vi "Configure.vi"(8 "error in":errorcluster, 10 "name":string="cCRDS", 11 "cCRDS in":refnum<class "cCRDS.lvclass">=refnum) -> (0 "error out":errorcluster, 3 "cCRDS out":refnum<class "cCRDS.lvclass">)   [LabVIEW 2015, in "cCRDS.lvclass"]
doc: "By far, the most complex of cCRDS VIs. This override of the Instrument Configure VI configures all signal input and output. The configuration is kicked off by calling the parent which sets up queues and names gives the class a unique name. Each CRDS class contains a CRDS Cell class which will encapsulate all of the defining characteristics of the discrete cell including how calculations are performed and the r factor (Optical Time Constant). In this case, each CRDS cell shares the same attributes aside from the wavelength of light used by the cavity.\n\nAfter the properties of the class are defined, the DAQmx tasks are configured. In this implementation, the CRDS utilizes two different laser types for light sources in the cavities: a dioed which requires a ring up time and a YAG which introduces light in pulses. Both laser sources (there are actually two diodes, red and blue, and one YAG, green) are fired using counter outputs. The YAG is synced with the diode counter by triggering the start of generation on the falling edge of the diode signal. On the laser acquisition side, the signal from the photodiodes is collected at a rate of 2.5 MS/s/ch using an S-series card. The acquisition signal is gated using the YAG counter signal which is tied to a counter on the S-series card across the PXI backplane using PXI_Trig0. The AI is acquired continuously clocking off of the other counter on the S-series card which is gated by the first counter.\n\nIn addition, the lasers and humidifier TECs are enabled and the humidifiers are set to their coldest temperature (corresponding to 5 V). All tasks are aggregated into a single array and started. If an error is thrown at config time, then the system will be shutdown."
uses:
  cCRDS.lvclass
  Data/cCRDS Data.lvclass
  Reusable/CRDS/Data/Cell/CRDS Cell Data.lvclass
  Reusable/CRDS/Main/CRDS.lvclass/CRDS.ctl
  Reusable/Instrument/Instrument.lvclass/Instrument.ctl
  Reusable/File IO/Class/File Observer.lvclass/File Observer.ctl
  cCRDS.lvclass/cCRDS.ctl
  Reusable/Instrument/state.ctl
  Reusable/Session APIs/File Access/Config Data/Config Data.lvclass
  Reusable/CRDS/Main/Read CRD RD Data Obs.vi
  Reusable/Instrument/Read Cfg Session.vi
  Reusable/File IO/Class/Accessors/Write Top Data Path.vi
  Reusable/File IO/Class/Accessors/Write File Prefix.vi
  Reusable/File IO/Class/Accessors/Write File Ext.vi
  Reusable/File IO/Class/Accessors/Write Max Size.vi
  Reusable/File IO/Class/Write SwitchonSize_.vi
  Reusable/File IO/Class/Write SwitchonDate_.vi
  Reusable/CRDS/Main/Write CRD RD Data Obs.vi
  Data Access/Write Laser Cfg.vi
  Reusable/CRDS/Data/Main/Write CellData.vi
  Reusable/CRDS/Main/Write Data.vi
  <vilib>/Utility/config.llb/Read Key (Double).vi
  Data Access/Write LF AI.vi
  Reusable/CRDS/Main/Read Cells.vi
  Reusable/CRDS/Cell/Write dt.vi
  Reusable/CRDS/Main/Write Cells.vi
  Reusable/File IO/Class/File Observer.lvclass
  <userlib>/_Session Fwk/Session - Root.lvclass
  Reusable/CRDS/Cell/CRDS Cell.lvclass
  Reusable/CRDS/Main/CRDS.lvclass
  Reusable/Instrument/Instrument.lvclass
  <vilib>/Utility/config.llb/NI_LVConfig.lvlib
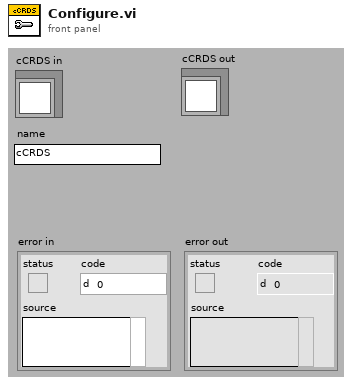
[diagram p1: front panel]
types:
  T1 = typedef "Session - Root.lvclass/Session Handle.ctl" = refnum<data-value>
  T2 = typedef "NI_LVConfig.lvlib/Config Data RefNum.ctl" = refnum<k1>
  T3 = typedef "Instrument.lvclass/state.ctl" = enum8{"Configure", "Acquire", "Wait", "Quit", "Handle Error", "NOOP"}
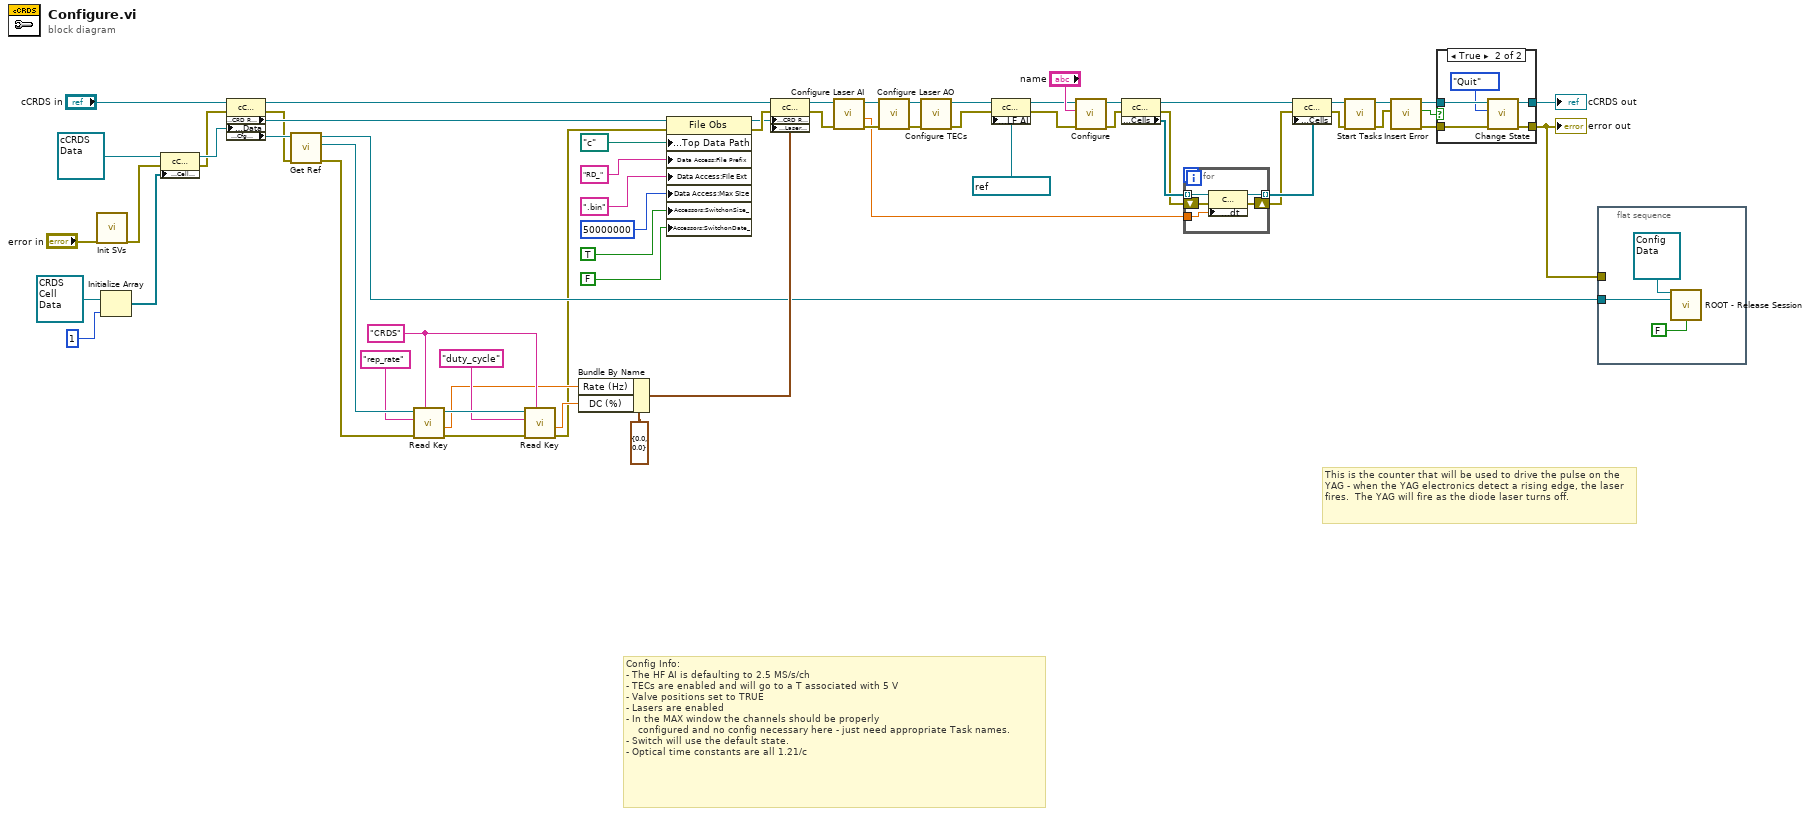
[diagram p0: block diagram]
diagram:
  w15 = "CRDS" ("section")
  # "Config Info:\n- The HF AI is defaulting to 2.5 MS/s/ch\n- TECs are enabled and will go to a T associated with 5 V\n- Valve positions set to TRUE\n- Lasers are enabled\n- In the MAX window the channels should be properly \n    configured and no config necessary here - just need appropriate Task names.\n- Switch will use the default state.\n- Optical time constants are all 1.21/c"
  # "This is the counter that will be used to drive the pulse on the YAG - when the YAG electronics detect a rising edge, the laser fires.  The YAG will fire as the diode laser turns off."
  n1 = call "Init SVs.vi"("error in"="error in") -> ("error out"=w6:errorcluster)  [unwired: 18 in]
  n2 = Initialize Array(refnum<class "CRDS Cell Data.lvclass"> refnum ("CRDS Cell"), 1 ("dimension size")) -> (w32:refnum<class "CRDS Cell Data.lvclass">[])
  n3 = property class="cCRDS Data"(reference=refnum<class "cCRDS Data.lvclass"> refnum ("cCRDS Data"), error in=w6, "Data Access:Cell Data"=w32) -> (reference out=w31:refnum<class "cCRDS Data.lvclass">, error out=w5:errorcluster)
  n4 = property class="cCRDS"(reference="cCRDS in", error in=w5, "Data Access:Data"=w31) -> (reference out=w41:refnum<class "cCRDS.lvclass">, error out=w4:errorcluster, "Accessors:CRD RD Data Obs"=w42:refnum<class "File Observer.lvclass">, "Accessors:Cfg Session"=w19:T1)
  n5 = call "Get Ref.vi"("error in"=w4, "Session Handle In"=w19) -> ("error out"=w3:errorcluster, "Ref"=w18:T2, "Session Handle Out"=w8:T1)  [unwired: 7 in]
  n6 = call-poly <vilib>:"Read Key.vi"("section"=w15, "error in (no error)"=w3, "key"="rep_rate", "refnum"=w18) -> ("error out"=w13:errorcluster, "value"=w11:dbl, "refnum out"=w16:T2)  [unwired: 4 in, 1 out]
  n7 = call-poly <vilib>:"Read Key.vi"("section"=w15, "error in (no error)"=w13, "key"="duty_cycle", "refnum"=w16) -> ("error out"=w1:errorcluster, "value"=w10:dbl)  [unwired: 4 in, 2 out]
  n8 = Bundle By Name(cluster=cluster{"Rate (Hz)":sgl, "DC (%)":sgl} {"Rate (Hz)"=0.0, "DC (%)"=0.0} ("Laser Cfg"), "Rate (Hz)"=w11, "DC (%)"=w10) -> (w9:cluster{"Rate (Hz)":sgl, "DC (%)":sgl})
  n9 = property class="File Obs"(reference=w42, error in=w1, "Data Access:Top Data Path"=path "c:/" ("RD Data Path"), "Data Access:File Prefix"="RD_" ("File Prefix"), "Data Access:File Ext"=".bin" ("File Prefix"), "Data Access:Max Size"=i64 50000000 ("Max Size"), "Accessors:SwitchonSize_"=TRUE ("SwitchonSize_"), "Accessors:SwitchonDate_"=FALSE ("SwitchonDate_")) -> (reference out=w39:refnum<class "File Observer.lvclass">, error out=w40:errorcluster)
  n10 = property class="cCRDS"(reference=w41, error in=w40, "Accessors:CRD RD Data Obs"=w39, "Accessors:Laser Cfg"=w9) -> (reference out=w38:refnum<class "cCRDS.lvclass">, error out=w37:errorcluster)
  n11 = call "Configure Laser AI.vi"("error in"=w37, "cCRDS in"=w38) -> ("error out"=w52:errorcluster, "dt"=w28:dbl, "cCRDS out"=w53:refnum<class "cCRDS.lvclass">)  [unwired: 7 in]
  n12 = call "Configure Laser AO.vi"("error in"=w52, "cCRDS in"=w53) -> ("error out"=w50:errorcluster, "cCRDS out"=w51:refnum<class "cCRDS.lvclass">)  [unwired: 8 in]
  n13 = call "Configure TECs.vi"("error in"=w50, "cCRDS in"=w51) -> ("error out"=w62:errorcluster, "cCRDS out"=w61:refnum<class "cCRDS.lvclass">)  [unwired: 8 in]
  n14 = property class="cCRDS"(reference=w61, error in=w62, "Accessors:LF AI"=refnum<k21> "CRD LFIO" ("Laser AI")) -> (reference out=w48:refnum<class "cCRDS.lvclass">, error out=w49:errorcluster)
  n15 = call-parent "Configure.vi"("error in"=w49, "name"="name", "CRDS in"=w48) -> ("error out"=w24:errorcluster, "CRDS out"=w30:refnum<class "cCRDS.lvclass">)  [unwired: 7 in]
  n16 = property class="cCRDS"(reference=w30, error in=w24) -> (reference out=w27:refnum<class "cCRDS.lvclass">, error out=w23:errorcluster, "Data Access:Cells"=w29:refnum<class "CRDS Cell.lvclass">[])
  n17 = for {
    tunnel: w29 -> [w68] mode=indexing
    tunnel: w28 -> [w67]
    tunnel: [w66] -> w26 mode=indexing
    shift-right: [w64] -> w22
    shift-left: w23 -> [w65]
    n18 = property class="CRDS Cell"(reference=w68, error in=w65, "Data Access:dt"=w67) -> (reference out=w66:refnum<class "CRDS Cell.lvclass">, error out=w64:errorcluster)
  }
  n19 = property class="cCRDS"(reference=w27, error in=w22, "Data Access:Cells"=w26) -> (reference out=w25:refnum<class "cCRDS.lvclass">, error out=w21:errorcluster)
  n20 = call "Start Tasks.vi"("error in"=w21, "cCRDS in"=w25) -> ("error out"=w59:errorcluster, "cCRDS out"=w58:refnum<class "cCRDS.lvclass">)  [unwired: 8 in]
  n21 = call "Insert Error.vi"("err"=w59, "Instrument in"=w58) -> ("error out"=w54:errorcluster, "error?"=w57:bool, "Instrument out"=w56:refnum<class "cCRDS.lvclass">)  [unwired: 7 in]
  n22 = case shown="True" w57 {
    tunnel: w56 -> [w70 w75]
    tunnel: [w70 w73] -> w55
    tunnel: [w69 w72] -> w2
    tunnel: w54 -> [w69 w71]
    frame False {
    }
    frame True {
      n23 = call "Change State.vi"("error in"=w71, "instr state"=state."Quit", "Instrument in"=w75) -> ("error out"=w72:errorcluster, "Instrument out"=w73:refnum<class "cCRDS.lvclass">)  [unwired: 7 in]
    }
  }
  "error out" <- w2
  "cCRDS out" <- w55
  n24 = flat-sequence {
    tunnel: w8 -> [w78]
    tunnel: w2 -> [_]
    frame #0 {
      n25 = call <userlib>:"ROOT - Release Session.vi"("OBJ - Session in"=refnum<class "Config Data.lvclass"> refnum ("Config Data"), "Session Handle in"=w78, "force destroy? (F)"=FALSE) -> ()  [unwired: 11 in, 2 out]
    }
  }
